vi "Queue Name - Error.vi"() -> (3 "Process Name":string="Error")   [LabVIEW 2016, in "System.lvlib"]
uses:
  System.lvlib
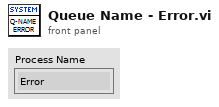
[diagram p1: front panel]
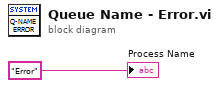
[diagram p0: block diagram]
diagram:
  "Process Name" <- "Error"
